vi "niRFSG Abort.vi"(0 "instrument handle":refnum<k15>, 11 "error in":errorcluster {"code" format="%.0x"}) -> (4 "instrument handle out":refnum<k15>, 15 "error out":errorcluster {"code" format="%.0x"})   [LabVIEW 2014]
doc: "Stops signal generation.\n\n<B>Supported Devices</B>: NI 5610/5611, NI 5644R/5645R/5646R, NI 5650/5651/5652/5654/5654 with NI 5696, NI 5670/5671/5672/5673/5673E, NI 5840"
uses:
  niRFSG.dll
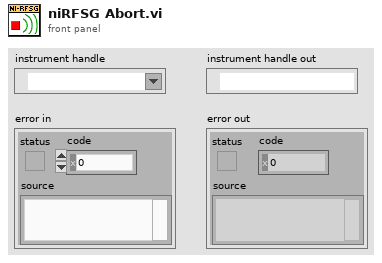
[diagram p1: front panel]
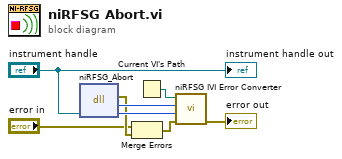
[diagram p0: block diagram]
diagram:
  n1 = dll-call lib="niRFSG**.*" fn="niRFSG_Abort"("instrument handle"="instrument handle") -> (error out=w2:errorcluster, "status"=w7:i32, "instrument handle"=w5:u32)  [unwired: 3 in, 1 out]
  n2 = Merge Errors("error in", w2) -> (w3:errorcluster)
  n3 = Current VI's Path() -> (path=w6:path)
  n4 = call "niRFSG IVI Error Converter.vi"("error in"=w3, "instrument handle"=w5, "IVI error code"=w7, "path to VI"=w6) -> ("error out"=→"error out":errorcluster)  [unwired: 7 out]
  "instrument handle out" <- "instrument handle"
